vi "ResetColor.vi"(8 "error in (no error)":errorcluster, 11 "FakedArray in":refnum<class "FakedArray.lvclass">) -> (0 "error out":errorcluster, 3 "FakedArray out":refnum<class "FakedArray.lvclass">)   [LabVIEW 2021, in "FakedArray.lvclass"]
uses:
  <resource>/plugins/NIIconEditor/Class/FakedArray/FakedArray.lvclass
  <resource>/plugins/NIIconEditor/Class/FakedArray/FakedArray.lvclass/FakedArray.ctl
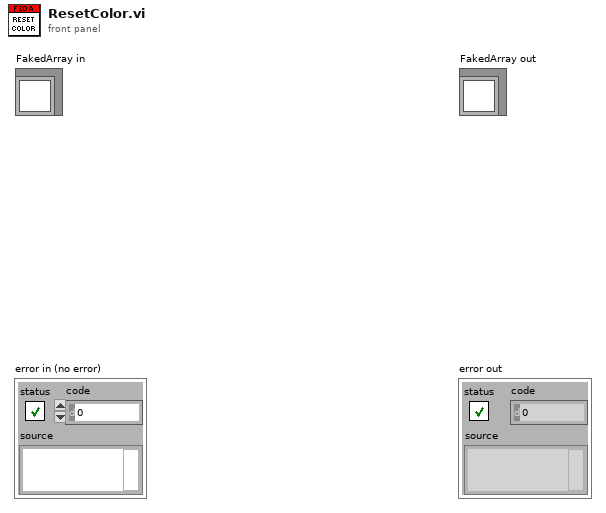
[diagram p1: front panel]
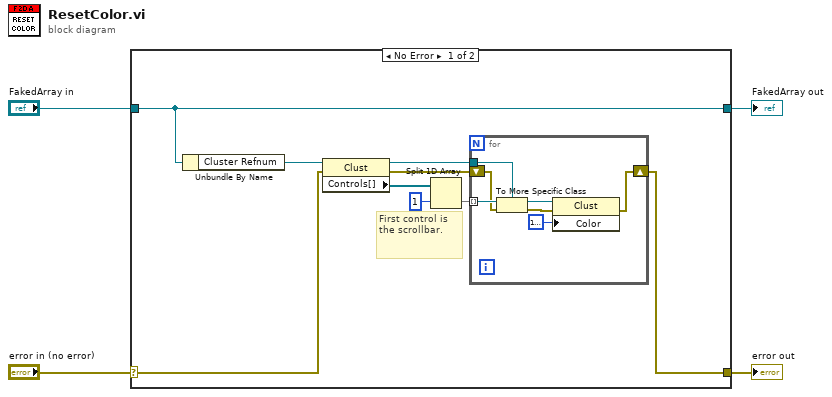
[diagram p0: block diagram]
diagram:
  n1 = case shown="No Error" "error in (no error)" {
    selector: "error in (no error)" -> [w6 w22]
    tunnel: [w5 w22] -> w3
    tunnel: [w13 w21] -> w1
    tunnel: "FakedArray in" -> [w13 w21]
    frame No Error {
      # "First control is the scrollbar."
      n2 = Unbundle By Name(w13) -> ("Cluster Refnum"=w12:refnum<vi>)
      n3 = property class="Clust"(reference=w12, error in=w6) -> (reference out=w8:refnum<vi>, error out=w7:errorcluster, "Controls[]"=w11:refnum<vi>[])
      n4 = Split 1D Array(array=w11, index=1) -> (second subarray=w9:refnum<vi>[])  [unwired: 1 out]
      n5 = for {
        tunnel: w9 -> [w20] mode=indexing
        tunnel: w8 -> [w18]
        shift-right: [w14] -> w5
        shift-left: w7 -> [w19]
        n6 = To More Specific Class(target class=w18, reference=w20, error in=w19) -> (specific class reference=w17:refnum<vi>, error out=w16:errorcluster)
        n7 = property class="Clust"(reference=w17, error in=w16, "Color"=u32 16777216) -> (error out=w14:errorcluster)  [unwired: 1 out]
      }
    }
    frame Error {
    }
  }
  "error out" <- w3
  "FakedArray out" <- w1
